vi "SetFrontPanelObjectControlValue.vi"(8 "error in (no error)":errorcluster, 9 "Control Name (\"\": Search by Type)":string, 10 "SMO":refnum<class "SMO.lvclass">, 11 "VI Ref In":refnum<vi>) -> (0 "error out":errorcluster, 3 "VI Ref Out":refnum<vi>)   [LabVIEW 2013, in "SMO.lvclass"]
doc: "Sets the FP control value of an LVClass control, whose type matches the specific type of object in <B>Object in</B> to the value of <B>Object in</B>.\n\n---------------------------------------------------------------\nJKI State Machine Objects™\nhttp://jki.net/state-machine-objects/\nCopyright (C) 2005-2015, JKI <info@jki.net>\nALL RIGHTS RESERVED"
uses:
  SMO.lvclass
  <vilib>/Utility/VariantDataType/VariantType.lvlib
panel:
  # "For instructions on how to use the JKI State Machine Objects, examples and video tutorials, visit:\nhttp://jki.net/state-machine-objects/\n\nJKI State Machine Objects™\nhttp://jki.net/state-machine-objects/\nCopyright (C) 2005-2015, JKI <info@jki.net>\nALL RIGHTS RESERVED"
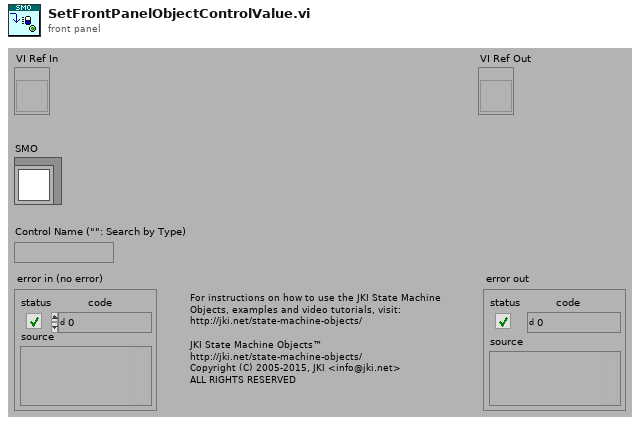
[diagram p1: front panel]
types:
  T1 = enum16{"Set Named Control", "Set Unamed Control", "Exit"}
  T2 = typedef "VariantType.lvlib/Type.ctl" = enum8{"Invalid Type", "Void", "I8", "I16", "I32", "I64", "U8", "U16", "U32", "U64", "Single Float", "Double Float", "Extended Float", "Single Complex", "Double Complex", "Extended Complex", "Enum U8", "Enum U16", "Enum U32", "Enum U64", "Single Float With Unit", "Double Float With Unit", "Extended Float With Unit", "Single Complex with Unit", "Double Complex with Unit", "Extended Complex with Unit", "Boolean", "String", "Path", "Picture", "Tag", "Array", "Cluster", "Variant", "LV Variant", "Waveform", "Timestamp", "Digital Waveform", "Digital Data", "ExpressData", "Refnum", "External Data", "VI", "Poly VI", "LabVIEW Class Instance", "Fixed Point"}
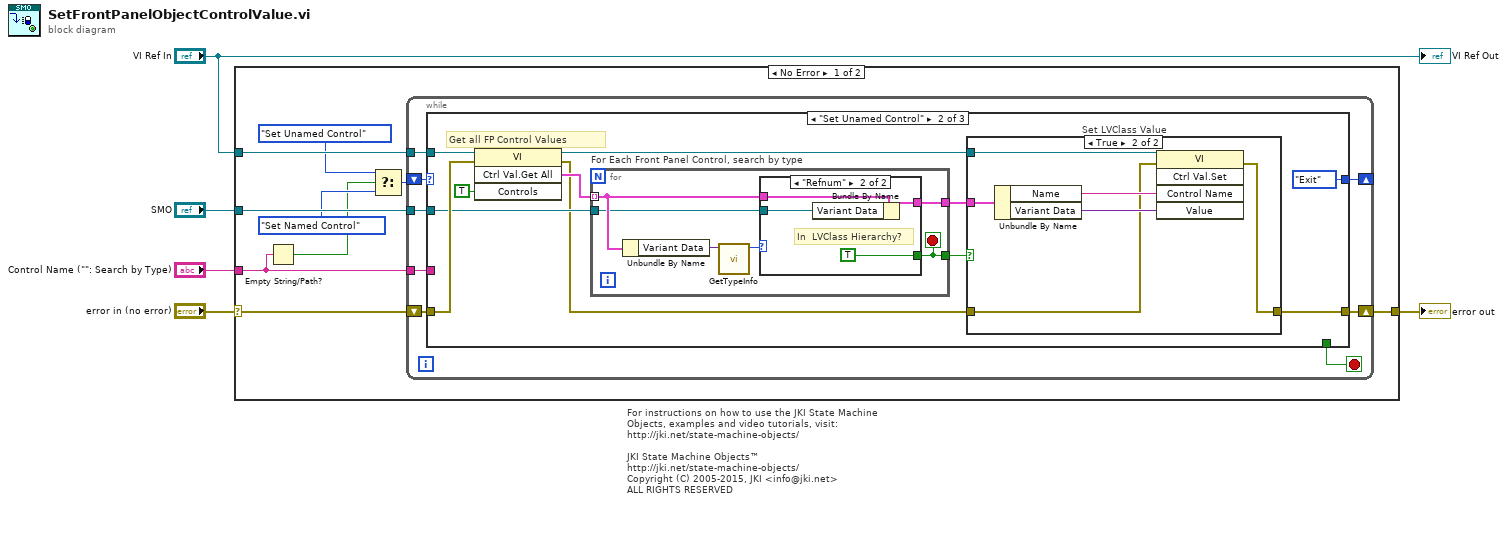
[diagram p0: block diagram]
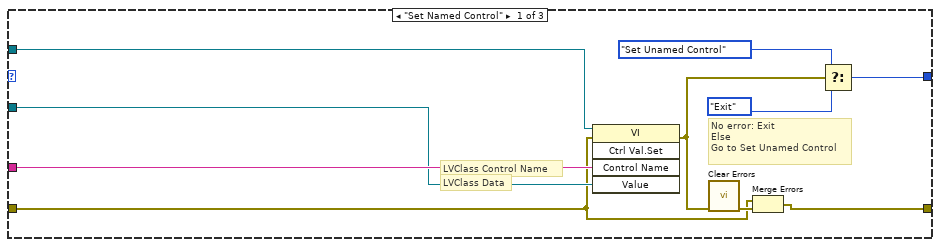
[diagram p2: hidden frame]
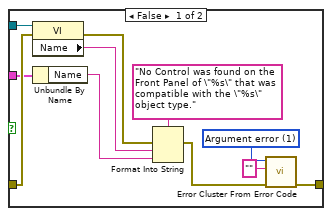
[diagram p3: hidden frame]
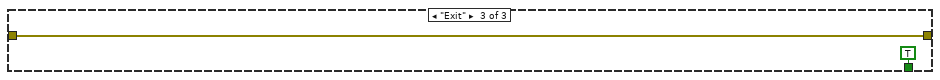
[diagram p5: hidden frame]
diagram:
  # "For instructions on how to use the JKI State Machine Objects, examples and video tutorials, visit:\nhttp://jki.net/state-machine-objects/\n\nJKI State Machine Objects™\nhttp://jki.net/state-machine-objects/\nCopyright (C) 2005-2015, JKI <info@jki.net>\nALL RIGHTS RESERVED"
  n1 = case shown="No Error" "error in (no error)" {
    selector: "error in (no error)" -> [w13 w74]
    tunnel: "SMO" -> [w11 _]
    tunnel: [w6 w74] -> w3
    tunnel: "VI Ref In" -> [w14 _]
    tunnel: "Control Name (\"\": Search by Type)" -> [w12 _]
    frame No Error {
      n2 = Empty String/Path?(string/path=w12) -> (empty?=w7:bool)
      n3 = Select(t=T1."Set Unamed Control", s=w7, f=T1."Set Named Control") -> (s? t:f=w10:T1)
      n4 = while {
        tunnel: w14 -> [w16]
        tunnel: w11 -> [w20]
        shift-right: [w18] -> w6
        shift-left: w13 -> [w21]
        shift-right: [w17] -> _
        shift-left: w10 -> [w22]
        tunnel: w12 -> [w19]
        stop <- w15 stop-if-true
        n5 = case shown="\"Set Unamed Control\"" w22 {
          tunnel: w21 -> [w23 w40 w72]
          tunnel: w20 -> [w31 w39 _]
          tunnel: w19 -> [w32 _ _]
          tunnel: [w24 w36 w72] -> w18
          tunnel: [w28 T1."Exit" _] -> w17
          tunnel: w16 -> [w26 w41 _]
          tunnel: [_ _ TRUE] -> w15
          frame "Set Named Control" {
            # "No error: Exit\nElse\nGo to Set Unamed Control"
            # "LVClass Control Name"
            # "LVClass Data"
            n6 = invoke class="VI" method="Ctrl Val.Set"(reference=w26, error in=w23, "Control Name"=w32, "Value"=w31) -> (error out=w30:errorcluster)  [unwired: 1 in, 4 out]
            n7 = call <vilib>:"Clear Errors.vi"("error in (no error)"=w30) -> ("error out"=w25:errorcluster)  [unwired: 6 in]
            n8 = Merge Errors(w23, w25) -> (w24:errorcluster)
            n9 = Select(t=T1."Set Unamed Control", s=w30, f=T1."Exit") -> (s? t:f=w28:T1)
          }
          frame "Set Unamed Control" {
            # "Get all FP Control Values"
            n10 = invoke class="VI" method="Ctrl Val.Get All"(reference=w41, error in=w40, "Controls"=TRUE) -> (reference out=w34:refnum<vi>, error out=w37:errorcluster, "Get All Control Values Variant"=w42:cluster{"Name":string, "Variant Data":variant}[])  [unwired: 1 in, 1 out]
            n11 = for "For Each Front Panel Control, search by type" {
              tunnel: w42 -> [w65] mode=indexing
              tunnel: [w64] -> w35
              tunnel: [w66] -> w33
              tunnel: w39 -> [w63]
              stop <- w66 stop-if-true
              n12 = Unbundle By Name(w65) -> ("Variant Data"=w62:variant)
              n13 = call <vilib>:"GetTypeInfo.vi"("Variant"=w62) -> ("Type Enum"=w61:T2)  [unwired: 6 in, 4 out]
              n14 = case shown="\"Refnum\"" w61 {
                tunnel: [_ TRUE] -> w66
                tunnel: w65 -> [w67 w71]
                tunnel: [w67 w70] -> w64
                tunnel: w63 -> [_ w68]
                frame Default {
                }
                frame "Refnum" {
                  # "In  LVClass Hierarchy?"
                  n15 = Bundle By Name(cluster=w71, "Variant Data"=w68) -> (w70:cluster{"Name":string, "Variant Data":variant})
                }
              }
            }
            n16 = case "Set LVClass Value" shown="True" w33 {
              tunnel: w35 -> [w45 w60]
              tunnel: [w54 w57] -> w36
              tunnel: w34 -> [w51 w56]
              tunnel: w37 -> [w46 w55]
              frame False {
                w53 = 1 items=["No error", "Argument error", "Memory is full", "Out of zone", "End of file", "File already open", "Generic file I/O error", "File not found", "File permission error", "Disk is full", "Duplicate path", "Too many files open", "System feature not enabled", "Resource file not found", "Cannot add resource", "Resource not found", "Image not found", "Image memory error", "Pen does not exist", "Config type invalid", "Config token not found", "Config parse error", "Config memory error", "Bad external code format", "Bad external code offset", "External code not present", "Null window", "Destroy window error", "Null menu", "Print aborted", "Bad print record", "Print driver error", "Windows error during printing", "Memory error during printing", "Print dialog error", "Generic print error", "Invalid device refnum", "Device not found", "Device parameter error", "Device unit error", "Cannot open device", "Device call aborted", "Generic error", "Cancelled by user", "Object ID too low", "Object ID too high", "Object not in heap", "Unknown heap", "Unknown object (invalid DefProc)", "Unknown object (DefProc not in table)", "Message out of range", "Invalid (null) method", "Unknown message", "Manager call not supported", "Bad address", "Network operation in progress", "Network operation timed out", "Connection is busy", "Network attribute not supported", "Network error", "Address in use", "System out of memory", "Connection aborted", "Connection refused", "Not connected", "Already connected", "Connection closed", "Initialization error (interapplication manager)", "Bad occurrence", "Wait on unbound occurrence handler", "Occurrence queue overflow", "Datalog type conflict", "Unused", "Unrecognized type (interapplication manager)", "Memory corrupt", "Failed to make temporary DLL", "Old CIN version", "Drag socket not found", "Failed to load drop-object", "Failed to register OLE object", "Failed to release OLE object", "Format specifier type mismatch", "Unknown format specifier", "Too few format specifiers", "Too many format specifiers", "Scan failed", "Newer CIN version", "Error converting to variant", "Runtime menu error", "Password tampered", "Variant attribute not found", "Incompatible variant data type", "Event data is not available", "Event Store is not present", "Occurrence is not found", "Event Queue is not created", "Event info is not available", "Refnum passed is NULL", "Error retrieving Class GUID", "Error retrieving CoClass GUID", "Error retrieving TypeLib GUID.", "Bad built application magic bytes.", "Specific driver is different from the specific driver associated with the Logical Name.", "There is no session opened to the class driver.", "Max Error", "MAX - Error with config objects", "MAX - Error loading configuration", "MAX - Group not supported"]
                n17 = property class="VI"(reference=w51, error in=w46) -> (error out=w48:errorcluster, "Name"=w50:string)  [unwired: 1 out]
                n18 = Unbundle By Name(w45) -> ("Name"=w44:string)
                n19 = Format Into String(format string="No Control was found on the Front Panel of \"%s\" that was compatible with the \"%s\" object type.", error in=w48, w50, w44) -> (error out=w47:errorcluster)  [unwired: 1 in, 1 out]
                n20 = call <vilib>:"Error Cluster From Error Code.vi"("error in (no error)"=w47, "error message (\"\")"="" ("error message (\"\")"), "error code (0)"=w53) -> ("error out"=w54:errorcluster)  [unwired: 1 in, 5 out]
              }
              frame True {
                n21 = Unbundle By Name(w60) -> ("Name"=w59:string, "Variant Data"=w58:variant)
                n22 = invoke class="VI" method="Ctrl Val.Set"(reference=w56, error in=w55, "Control Name"=w59, "Value"=w58) -> (error out=w57:errorcluster)  [unwired: 1 in, 4 out]
              }
            }
          }
          frame "Exit" {
          }
        }
      }
    }
    frame Error {
    }
  }
  "error out" <- w3
  "VI Ref Out" <- "VI Ref In"
